vi "Timer.vi"(1 "Seconds (string)":string) -> (0 "Done":bool)   [LabVIEW 2013]
doc: "A timer. Converts a string parameter into a number to be used as the time."
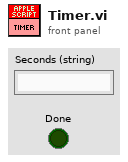
[diagram p1: front panel]
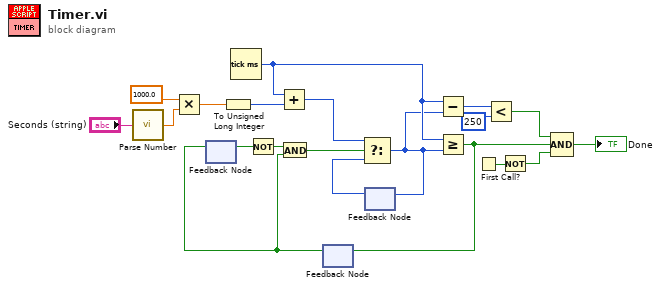
[diagram p0: block diagram]
diagram:
  n1 = call "Parse Number.vi"("String"="Seconds (string)") -> ("Number"=w4:dbl)
  n2 = Multiply(x=1000.0, y=w4) -> (x*y=w14:dbl)
  n3 = feedback #1() -> (w17:bool)  [unwired: 1 in]
  n4 = To Unsigned Long Integer(number=w14) -> (unsigned 32bit integer=w13:u32)
  n5 = Tick Count (ms)() -> (millisecond timer value=w3:u32)
  n6 = Not(x=w17) -> (.not. x?=w16:bool)
  n7 = Add(x=w3, y=w13) -> (x+y=w20:u32)
  n8 = feedback #2() -> (w12:bool)  [unwired: 1 in]
  n9 = feedback-in #1(w12) -> ()
  n10 = And(x=w16, y=w12) -> (x .and. y?=w18:bool)
  n11 = feedback #3() -> (w19:u32)  [unwired: 1 in]
  n12 = Select(t=w20, s=w18, f=w19) -> (s? t:f=w2:u32)
  n13 = feedback-in #3(w2) -> ()
  n14 = Subtract(x=w3, y=w2) -> (x-y=w10:u32)
  n15 = Greater Or Equal?(x=w3, y=w2) -> (x >= y?=w8:bool)
  n16 = feedback-in #2(w8) -> ()
  n17 = First Call?() -> (First Call?: T/F=w11:bool)
  n18 = Less?(x=w10, y=u32 250) -> (x < y?=w7:bool)
  n19 = Not(x=w11) -> (.not. x?=w1:bool)
  n20 = Compound Arithmetic op=AND(w7, w8, w1) -> (→"Done":bool)
